vi "Line and Page Break Constant Shell.vi"   [LabVIEW 2020]
doc: "Defines line and page break attributes of a specified range within a document."
uses:
  <vilib>/addons/_office/NI_ReportGenerationToolkit.lvlib
types:
  T1 = cluster{"Widow/orphan ctrl":u16, "Keeps lines together":u16, "Keep with next":u16, "Page break before":u16, "Suppress line numbers":u16, "Don't hyphenate":u16}
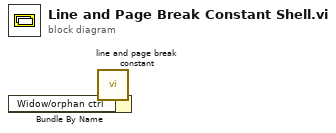
[diagram p0: block diagram]
diagram:
  n1 = call <vilib>:"line and page break constant.vi"() -> ("line and page breaks"=w1:T1)
  n2 = Bundle By Name(cluster=w1) -> ()  [unwired: 1 in, 1 out]
